vi "e.gate HighSpeedPort Get File - Read FileSize.vi"(7 "Timeout (ms) [1000]":i32=1000, 8 "error in (no error)":errorcluster, 10 "File or relative Path":string, 11 "Configuration in":T1) -> (0 "error out":errorcluster, 2 "data out (string)":string, 3 "Configuration out":T1)   [LabVIEW 2016]
uses:
  e.gate Configuration.ctl
  e.gate Channel Data.ctl
  e.gate Data Type.ctl
  e.gate Protocol Type.ctl
  e.gate Module  Data.ctl
  e.gateHSP_DLLhandle.ctl
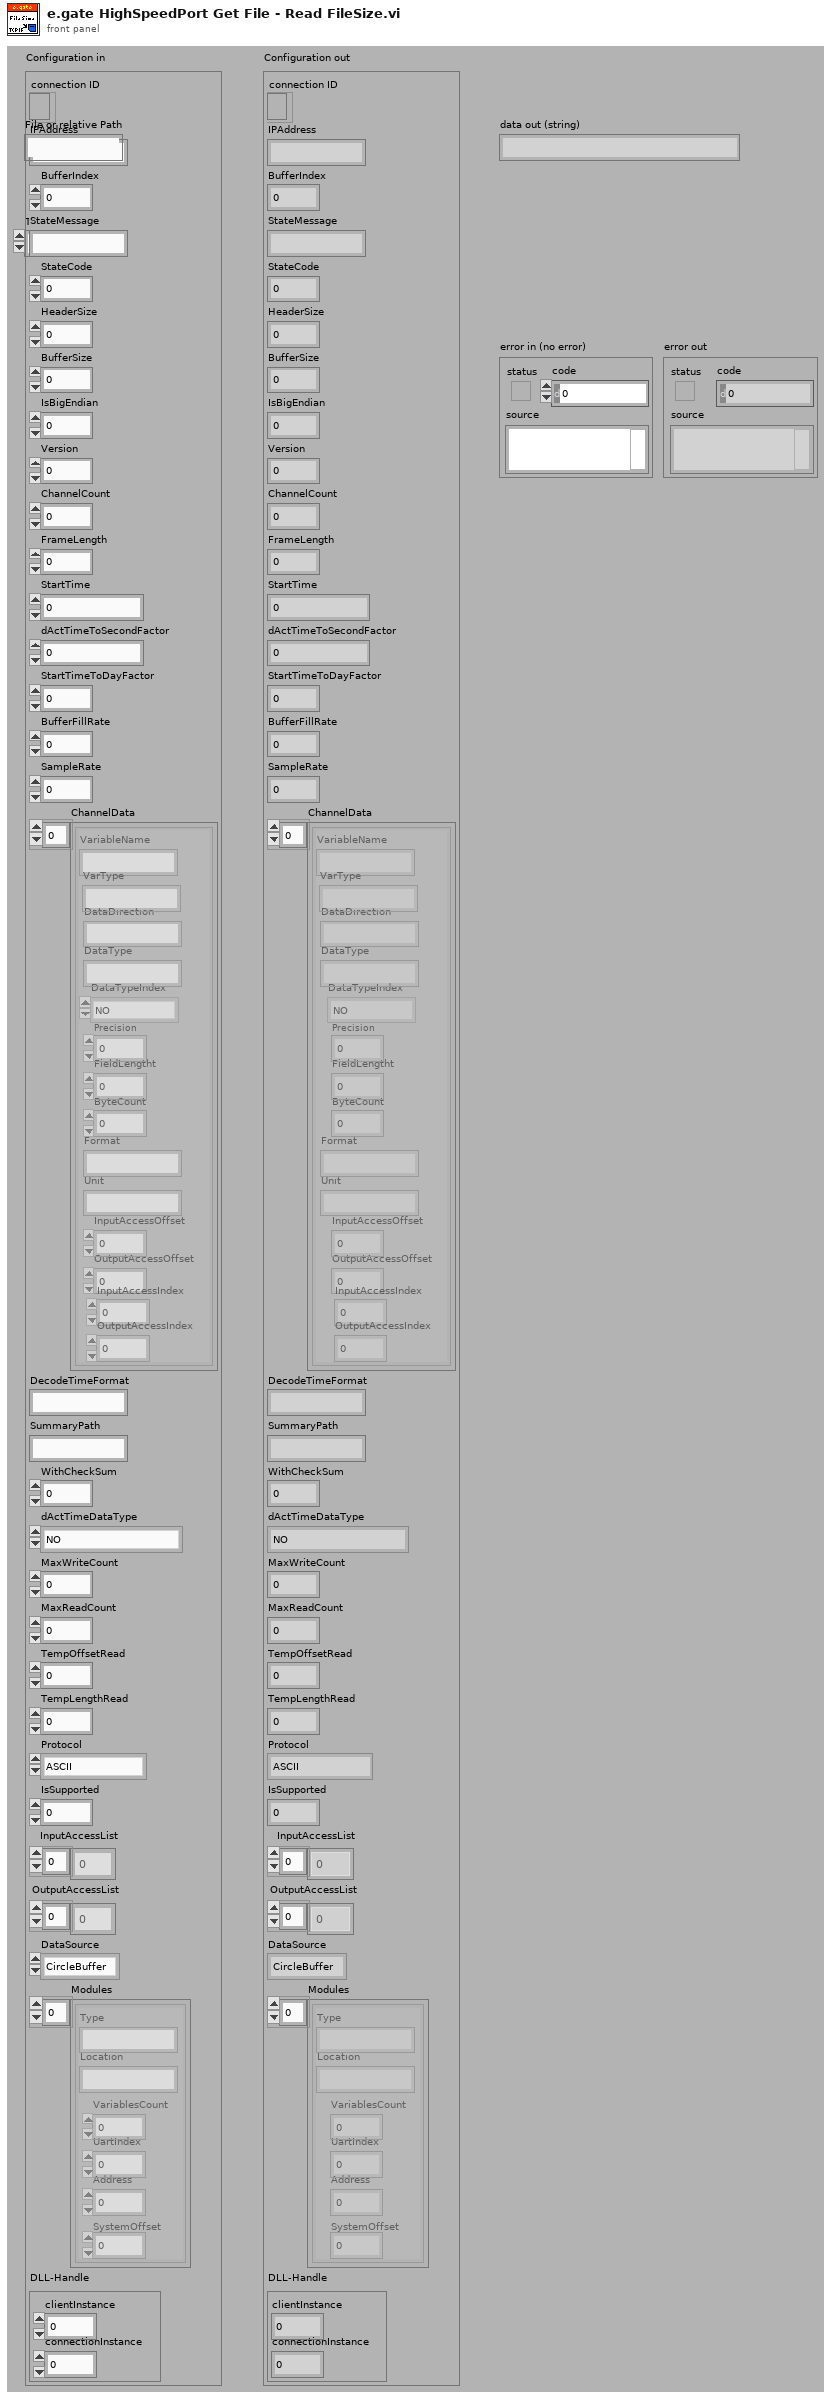
[diagram p1: front panel]
types:
  T1 = typedef "e.gate Configuration.ctl" = cluster{"connection ID":refnum<k5>, "IPAddress":string, "BufferIndex":i32, "StateMessage":string, "StateCode":i8, "HeaderSize":i32, "BufferSize":i32, "IsBigEndian":i32, "Version":i32, "ChannelCount":i32, "FrameLength":i32, "StartTime":dbl, "dActTimeToSecondFactor":dbl, "StartTimeToDayFactor":dbl, "BufferFillRate":dbl, "SampleRate":dbl, "ChannelData":T2[], "DecodeTimeFormat":string, "SummaryPath":string, "WithCheckSum":i32, "dActTimeDataType":T3, "MaxWriteCount":i32, "MaxReadCount":i32, "TempOffsetRead":i32, "TempLengthRead":i32, "Protocol":T4, "IsSupported":i32, "InputAccessList":i32[], "OutputAccessList":i32[], "DataSource":enum16{"CircleBuffer", "test.con Logger", "test.con Archive"}, "Modules":T5[], "DLL-Handle":T6}
  T2 = typedef "e.gate Channel Data.ctl" = cluster{"VariableName":string, "DataDirection":string, "DataType":string, "DataTypeIndex":T3, "Precision":i16, "FieldLengtht":i16, "ByteCount":i32, "Format":string, "Unit":string, "InputAccessOffset":i32, "OutputAccessOffset":i16, "InputAccessIndex":i16, "OutputAccessIndex":i16, "VarType":string}
  T3 = typedef "e.gate Data Type.ctl" = enum16{"NO", "BOOL", "SINT8", "USINT8", "SINT16", "USINT16", "SINT32", "USINT32", "FLOAT", "SET8", "SET16", "SET32", "DOUBLE", "SINT64", "USINT64", "SET64"}
  T4 = typedef "e.gate Protocol Type.ctl" = enum16{"ASCII", "HighspeedPort Online", "HighspeedPort Buffer", "eGateHighspeedPortDLL "}
  T5 = typedef "e.gate Module  Data.ctl" = cluster{"Type":string, "Location":string, "VariablesCount":i16, "UartIndex":i16, "Address":i16, "SystemOffset":i16}
  T6 = typedef "e.gateHSP_DLLhandle.ctl" = cluster{"clientInstance":i32, "connectionInstance":i32}
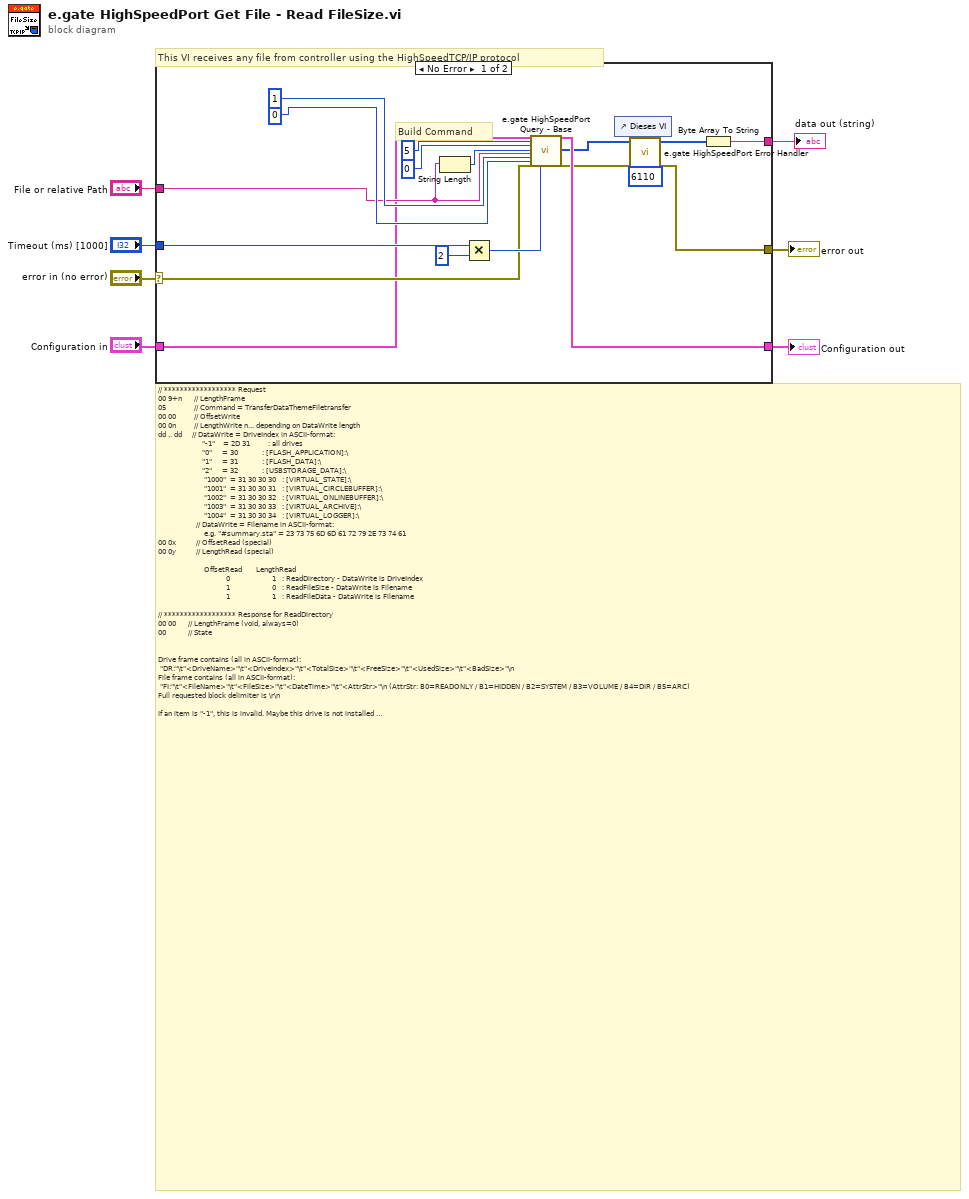
[diagram p0: block diagram]
diagram:
  # "// ****************** Request\n00 9+n\t\t\t\t\t\t// LengthFrame\n05\t\t\t\t\t\t\t       // Command = TransferDataThemeFiletransfer\n00 00\t\t\t\t   \t\t// OffsetWrite\n00 0n\t\t\t\t\t   \t// LengthWrite n... depending on DataWrite length\ndd .. dd\t\t\t\t\t// DataWrite = DriveIndex in ASCII-format:\n\t\t\t\t\t\t\t              \t\"-1\"    = 2D 31         : all drives\n\t\t\t\t\t\t              \t\t\"0\"     = 30            : [FLASH_APPLICATION]:\\\n\t\t\t\t\t\t\t              \t\"1\"     = 31            : [FLASH_DATA]:\\\n\t\t\t              \t\t\t\t\t\"2\"     = 32            : [USBSTORAGE_DATA]:\\\n\t\t\t\t\t\t               \t\t\"1000\"  = 31 30 30 30   : [VIRTUAL_STATE]:\\\n\t\t\t\t\t\t\t               \t\"1001\"  = 31 30 30 31   : [VIRTUAL_CIRCLEBUFFER]:\\\n\t\t\t\t\t\t\t               \t\"1002\"  = 31 30 30 32   : [VIRTUAL_ONLINEBUFFER]:\\\n\t\t\t\t\t\t               \t\t\"1003\"  = 31 30 30 33   : [VIRTUAL_ARCHIVE]:\\\n\t\t\t\t\t\t               \t\t\"1004\"  = 31 30 30 34   : [VIRTUAL_LOGGER]:\\\n\t\t\t\t\t\t            \t// DataWrite = Filename in ASCII-format:\n\t\t\t\t\t\t\t               \te.g. \"#summary.sta\" = 23 73 75 6D 6D 61 72 79 2E 73 74 61\n00 0x\t\t\t\t\t\t    // OffsetRead (special)\n00 0y\t\t\t\t\t\t    // LengthRead (special)\n\n\t\t\t\t\t\t\t\t               OffsetRead      \tLengthRead\n\t\t\t\t\t\t\t                          \t0\t                  \t\t1\t\t\t: ReadDirectory - DataWrite is DriveIndex\n\t\t\t\t\t\t\t                          \t1\t\t                  \t0\t\t\t: ReadFileSize - DataWrite is Filename\n\t\t\t\t\t\t\t                          \t1\t\t\t                  1\t\t\t: ReadFileData - DataWrite is Filename\n\n// ****************** Response for ReadDirectory\n00 00\t\t\t\t\t\t// LengthFrame (void, always=0)\n00\t\t\t\t\t    \t\t// State\n\n\nDrive frame contains (all in ASCII-format):\n\t\"DR:\"\\t\"<DriveName>\"\\t\"<DriveIndex>\"\\t\"<TotalSize>\"\\t\"<FreeSize>\"\\t\"<UsedSize>\"\\t\"<BadSize>\"\\n\nFile frame contains (all in ASCII-format):\n\t\"FI:\"\\t\"<FileName>\"\\t\"<FileSize>\"\\t\"<DateTime>\"\\t\"<AttrStr>\"\\n\t(AttrStr: B0=READONLY / B1=HIDDEN / B2=SYSTEM / B3=VOLUME / B4=DIR / B5=ARC)\nFull requested block delimiter is \\r\\n\n\nIf an item is \"-1\", this is invalid. Maybe this drive is not installed or parameter is not available there !!!\n\ne.g. ReadDirectory of DriveIndex=0:\n\\x00\\x00\\x00\nDR:\\t[FLASH_APPLICATION]:\\\\t0\\t7077888\\t4878336\\t2199552\\t0\\n\nFI:\\tecpu01.bin\\t1764336\\t2008-03-11\\t10:51:40\\t0020\\n\nFI:\\tecpu01.ini\\t495\\t1980-01-01\\t12:00:00\\t0020\\n\nFI:\\tconfig.sys\\t219\\t1980-01-01\\t12:00:00\\t0020\\n\nFI:\\tfpga.bit\\t403014\\t1980-01-01\\t12:00:00\\t0020\\n\nFI:\\tftp_lic.cnf\\t538\\t2008-02-26\\t15:43:42\\t0020\\n\nFI:\\tmaster.gcf\t10750\\t2008-02-26\\t15:43:50\\t0020\\n\nFI:\\tself.ini\\t78\\t2008-03-11 09:27:36\\t0020\\n\\r\\n\n\n// ****************** Response for ReadFileSize\n00 1+n\t\t\t\t\t\t// LengthFrame\n00\t\t\t\t\t\t       \t// State\ndd .. dd\t\t\t\t\t// DataRead: Size of file in ASCII-format with length n\n\n// ****************** Response for ReadFileData\n00 1+n\t\t\t\t\t\t// LengthFrame\n00\t\t\t\t\t\t       \t// State\ndd .. dd\t\t\t\t\t// DataRead: Content of file with length n\n\n\nATTENTION: If LengthFrame is 0xFFFF, an ExtendedLengthFrame element with 4 bytes is inserted after LF LF, to make possible,\n\tto transfer more than 65534 bytes of data !!!"
  # "This VI receives any file from controller using the HighSpeedTCP/IP protocol"
  n1 = case shown="No Error" "error in (no error)" {
    selector: "error in (no error)" -> [w20 w27]
    tunnel: [w15 w28] -> w6
    tunnel: "Configuration in" -> [w16 w28]
    tunnel: [w8 w27] -> w3
    tunnel: "Timeout (ms) [1000]" -> [w26 _]
    tunnel: "File or relative Path" -> [w17 _]
    tunnel: [w9 _] -> w1
    frame No Error {
      # "Build Command"
      n2 = String Length(string=w17) -> (length=w21:i32)
      n3 = Multiply(x=w26, y=2) -> (x*y=w24:i32)
      n4 = call "e.gate HighSpeedPort Query - Base.vi"("e.gate Configuration in"=w16, "Command"=5, "OffsetWrite"=0 ("Command"), "LengthWrite"=w21, "DataWrite"=w17, "OffsetRead"=1 ("Command"), "LengthRead"=0 ("Command"), "error in (no error)"=w20, "Timeout (1000)"=w24) -> ("e.gate Configuration out"=w15:T1, "Data (out binary)"=w12:u8[], "error out"=w11:errorcluster)  [unwired: 1 in, 15 out]
      n5 = control-ref of="Dieses VI"() -> (w13:refnum<vi>)
      n6 = call "e.gate HighSpeedPort Error Handler.vi"("error code start index"=6110, "VI reference"=w13, "error in (no error)"=w11, "binary data in"=w12) -> ("error out"=w8:errorcluster, "binary out"=w10:u8[])  [unwired: 6 out]
      n7 = Byte Array To String(unsigned byte array=w10) -> (string=w9:string)
    }
    frame Error {
    }
  }
  "Configuration out" <- w6
  "error out" <- w3
  "data out (string)" <- w1
